vi "Scroll into View.vi"() -> ()   [LabVIEW 2020, in "Array Example.lvlib"]
uses:
  Array Example.lvlib
  Element B/Element B.lvclass
  C:/dev/lv20CE/lv-oopanel/Examples/Array/Element Base/Element Base.lvclass
  Element A/Element A.lvclass
  Element Base/Element Base.lvclass
  C:/dev/lv20CE/lv-oopanel/OOPanel/ArrayPanel/ArrayPanel.lvclass
  OOPanel/ArrayManager/ArrayManager.lvclass
panel:
  in  "Scroll To":bool
  in  "Index":i32
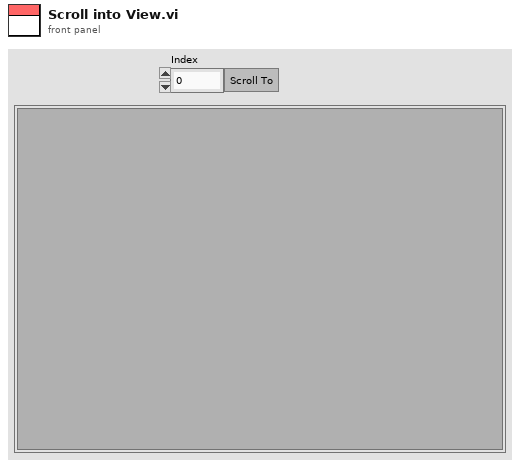
[diagram p1: front panel]
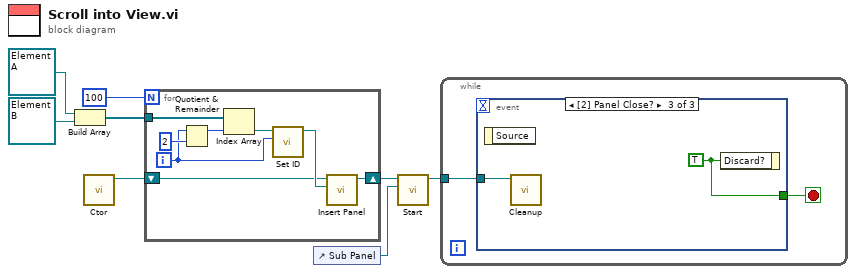
[diagram p0: block diagram]
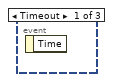
[diagram p2: hidden frame]
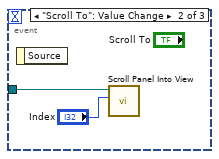
[diagram p3: hidden frame]
diagram:
  n1 = Build Array(refnum<class "Element A.lvclass"> refnum ("Array Example.lvlib:Element A.lvclass"), refnum<class "Element B.lvclass"> refnum ("Array Example.lvlib:Element B.lvclass")) -> (w6:refnum<class "Element Base.lvclass">[])
  n2 = call "Ctor.vi"() -> ("PanelArray"=w8:refnum<class "ArrayManager.lvclass">)  [unwired: 10 in, 1 out]
  n3 = for {
    N: 100 -> [_]
    tunnel: w6 -> [w15]
    shift-right: [w12] -> w4
    shift-left: w8 -> [w9]
    i -> [w13]
    n4 = Quotient & Remainder(x=w13, y=2) -> (x-y*floor(x/y)=w14:i32)  [unwired: 1 out]
    n5 = Index Array(array=w15, index=w14) -> (element=w11:refnum<class "Element Base.lvclass">)
    n6 = call "Set ID.vi"("ID"=w13, "Element Base in"=w11) -> ("Element Base out"=w10:refnum<class "Element Base.lvclass">)  [unwired: 8 in, 1 out]
    n7 = call "Insert Panel.vi"("Panel/Type"=w10, "PanelArray in"=w9) -> ("PanelArray out"=w12:refnum<class "ArrayManager.lvclass">)  [unwired: 7 in, 2 out]
  }
  n8 = control-ref of="Sub Panel"() -> (w3:refnum<vi>)
  n9 = call "Start.vi"("Container"=w3, "ArrayManager in"=w4) -> ("ArrayManager out"=w1:refnum<class "ArrayManager.lvclass">)  [unwired: 8 in, 1 out]
  n10 = while {
    tunnel: w1 -> [w18]
    stop <- w17 stop-if-true
    n11 = event shown="[2] Panel Close?" {
      selector: _ -> [_ _ _]
      dyn-events: _ -> [_ _ _]
      timeout: _ -> [_ _ _]
      tunnel: w18 -> [_ w20 w21]
      tunnel: [_ _ w22] -> w17
      event Timeout {
        n12 = event-data() -> ()  [unwired: 1 in, 1 out]
      }
      event "Scroll To": Value Change {
        n13 = event-data() -> ()  [unwired: 1 in, 1 out]
        n14 = call "Scroll Panel Into View.vi"("Panel Index"="Index", "ArrayManager in"=w20) -> ()  [unwired: 8 in, 2 out]
      }
      event Panel Close? {
        w22 = TRUE ("Discard?")
        n15 = event-data() -> ()  [unwired: 1 in, 1 out]
        n16 = call "Cleanup.vi"("PanelArray in"=w21) -> ()  [unwired: 10 in, 1 out]
        n17 = event-data("Discard?"=w22) -> ()  [unwired: 1 in, 1 out]
      }
    }
  }
